vi "TCP Connection.vi"(7 "phase shift array":i32[](array[numeric]), 8 "error in (no error)":errorcluster, 9 "timeout ms (60000)":i32, 10 "remote port or service name":u16=1112, 11 "address":string) -> (0 "error out":errorcluster, 3 "failure setting of phases":i32[](array[numeric]))   [LabVIEW 2014]
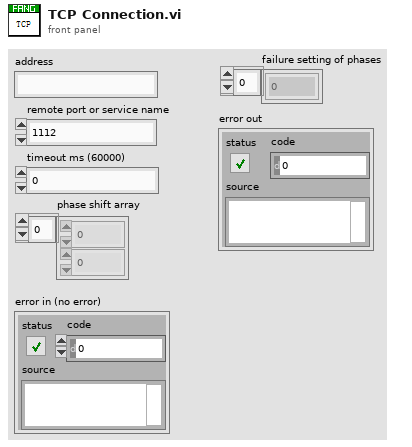
[diagram p1: front panel]
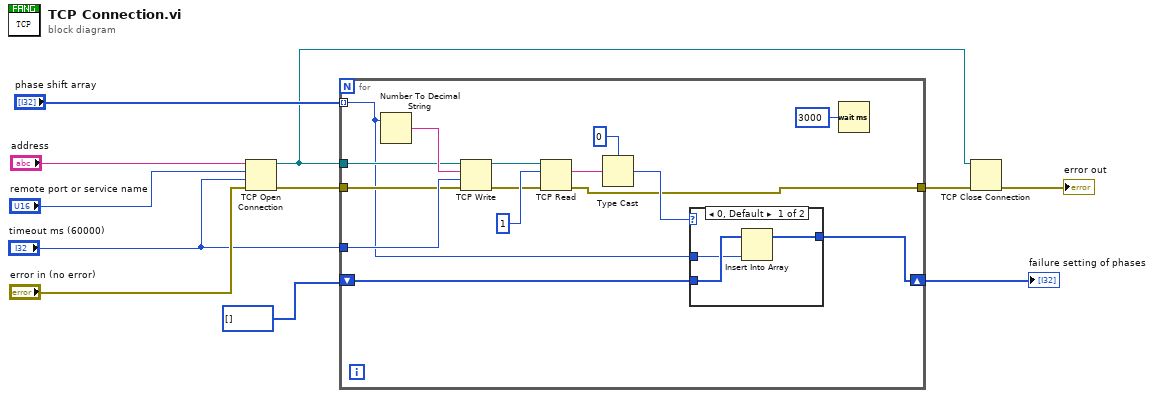
[diagram p0: block diagram]
diagram:
  n1 = TCP Open Connection(address="address", remote port or service name="remote port or service name", timeout ms (60000)="timeout ms (60000)", error in (no error)="error in (no error)") -> (connection ID=w3:refnum<k5>, error out=w7:errorcluster)  [unwired: 1 in]
  n2 = for {
    tunnel: "phase shift array" -> [w16] mode=indexing
    tunnel: w3 -> [w25]
    tunnel: w7 -> [w23]
    tunnel: "timeout ms (60000)" -> [w24]
    shift-right: [w15] -> w5
    shift-left: i32[] [] -> [w17]
    tunnel: [w13] -> w4
    n3 = Number To Decimal String(number=w16) -> (decimal integer string=w26:string)  [unwired: 1 in]
    n4 = TCP Write(connection ID=w25, data in=w26, error in (no error)=w23, 9:w24) -> (connection ID out=w22:refnum<k5>, error out=w14:errorcluster)  [unwired: 1 out]
    n5 = TCP Read(connection ID=w22, bytes to read=1, error in (no error)=w14) -> (data out=w20:string, error out=w13:errorcluster)  [unwired: 2 in, 1 out]
    n6 = Type Cast(type=i8 0, x=w20) -> (*(type *) &x=w18:i8)
    n7 = case shown="0, Default" w18 {
      tunnel: w17 -> [w29 w30]
      tunnel: w16 -> [w28 _]
      tunnel: [w27 w30] -> w15
      frame 0, Default {
        n8 = Insert Into Array(array=w29, new element=w28) -> (w27:i32[])  [unwired: 1 in]
      }
      frame 1 {
      }
    }
    n9 = Wait (ms)(milliseconds to wait=u32 3000) -> ()  [unwired: 1 out]
  }
  "failure setting of phases" <- w5
  n10 = TCP Close Connection(connection ID=w3, error in (no error)=w4) -> (error out=→"error out":errorcluster)  [unwired: 1 in, 1 out]
